vi "Open OPC UA Connection.vi"(8 "error in (no error)":errorcluster, 10 "OPC UA configuration":refnum<class "OPC UA Client configuration.lvclass">, 11 "OPC UA runtime in":refnum<class "OPC UA Client runtime.lvclass">) -> (0 "error out":errorcluster, 3 "OPC UA runtime out":refnum<class "OPC UA Client runtime.lvclass">)   [LabVIEW 2013, in "OPC UA Client runtime.lvclass"]
doc: "Opens connection to an OPC UA Client"
uses:
  OPC UA Client runtime.lvclass
  configuration/OPC UA Client configuration.lvclass
  configuration/OPC UA Client configuration.lvclass/OPC UA Client configuration.ctl
  OPC UA Client runtime.lvclass/OPC UA Client runtime.ctl
  configuration/Read Connection Configuration.vi
  <vilib>/opcua/NI OPC UA Client.lvlib
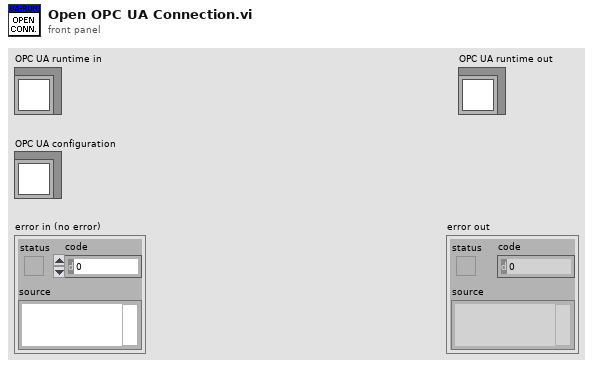
[diagram p1: front panel]
types:
  T1 = typedef "OPC UA Client configuration.lvclass/Client Connection Configuration.ctl" = cluster{"Server Certificates":cluster{"Relative Path?":bool, "Server Paths":string[]}, "Client Certificates":cluster{"Relative Path?":bool, "Client Path":string}, "Client Configuration":cluster{"Server Endpoint URL":string, "Security Policy":cluster{"Message Mode":enum16{"None", "Sign", "Sign and Encrypt"}, "Security":enum16{"Basic256", "Basic128Rsa15"}}, "Username/Password":cluster{"Username":string, "Password":string}}}
  T2 = cluster{"Message Mode":enum16{"None", "Sign", "Sign and Encrypt"}, "Security":enum16{"Basic256", "Basic128Rsa15"}}
  T3 = cluster{"Relative Path?":bool, "Client Path":string}
  T4 = cluster{"Relative Path?":bool, "Server Paths":string[]}
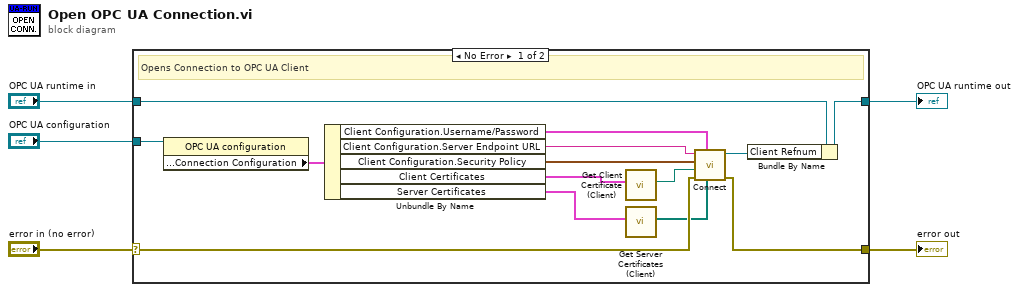
[diagram p0: block diagram]
diagram:
  n1 = case shown="No Error" "error in (no error)" {
    selector: "error in (no error)" -> [w17 w21]
    tunnel: [w16 w21] -> w4
    tunnel: [w18 w20] -> w2
    tunnel: "OPC UA runtime in" -> [w19 w20]
    tunnel: "OPC UA configuration" -> [w7 _]
    frame No Error {
      # "Opens Connection to OPC UA Client"
      n2 = property class="OPC UA configuration"(reference=w7) -> ("Customize:Properties:Connection Configuration"=w6:T1)  [unwired: 1 in, 2 out]
      n3 = Unbundle By Name(w6) -> ("Client Configuration.Username/Password"=w14:cluster{"Username":string, "Password":string}, "Client Configuration.Server Endpoint URL"=w13:string, "Client Configuration.Security Policy"=w12:T2, "Client Certificates"=w11:T3, "Server Certificates"=w9:T4)
      n4 = call "Get Client Certificate (Client).vi"("Client Certificates"=w11) -> ("client certificate file"=w10:path)  [unwired: 10 in]
      n5 = call "Get Server Certificates (Client).vi"("Server Certificates"=w9) -> ("trusted server certificates"=w8:path[])  [unwired: 10 in]
      n6 = call <vilib>:"Connect.vi"("trusted server certificates"=w8, "username/password"=w14, "error in (no error)"=w17, "client certificate file"=w10, "security policy"=w12, "server endpoint URL"=w13) -> ("error out"=w16:errorcluster, "OPC UA client refnum out"=w15:refnum<k21>)  [unwired: 3 in, 1 out]
      n7 = Bundle By Name(cluster=w19, "Client Refnum"=w15) -> (w18:refnum<class "OPC UA Client runtime.lvclass">)
    }
    frame Error {
    }
  }
  "error out" <- w4
  "OPC UA runtime out" <- w2
